vi "__keysight_volatile_test.vi"() -> ()   [LabVIEW 2013]
uses:
  <vilib>/Analysis/NI_AALBase.lvlib
panel:
  out "Numeric":i32
  in  "Frequency Parameters":T1={"Coupling"=TRUE, "Frequency 2 (MHz)"=2.0, "Frequency 1 (MHz)"=2.0} {"Frequency 1 (MHz)" min=0.0 max=14.5; "Frequency 2 (MHz)" min=0.0 max=14.5}
  in  "Array to Binary Block Format 2":dbl[](array[numeric])
  out "concatenated string":string
  out "Waveform Graph":dbl[](graph)
  in  "Pulse Width":i32=1
  in  "N-per-period":i32=20001
  in  "GPIB address of Pulse generator":string="10"
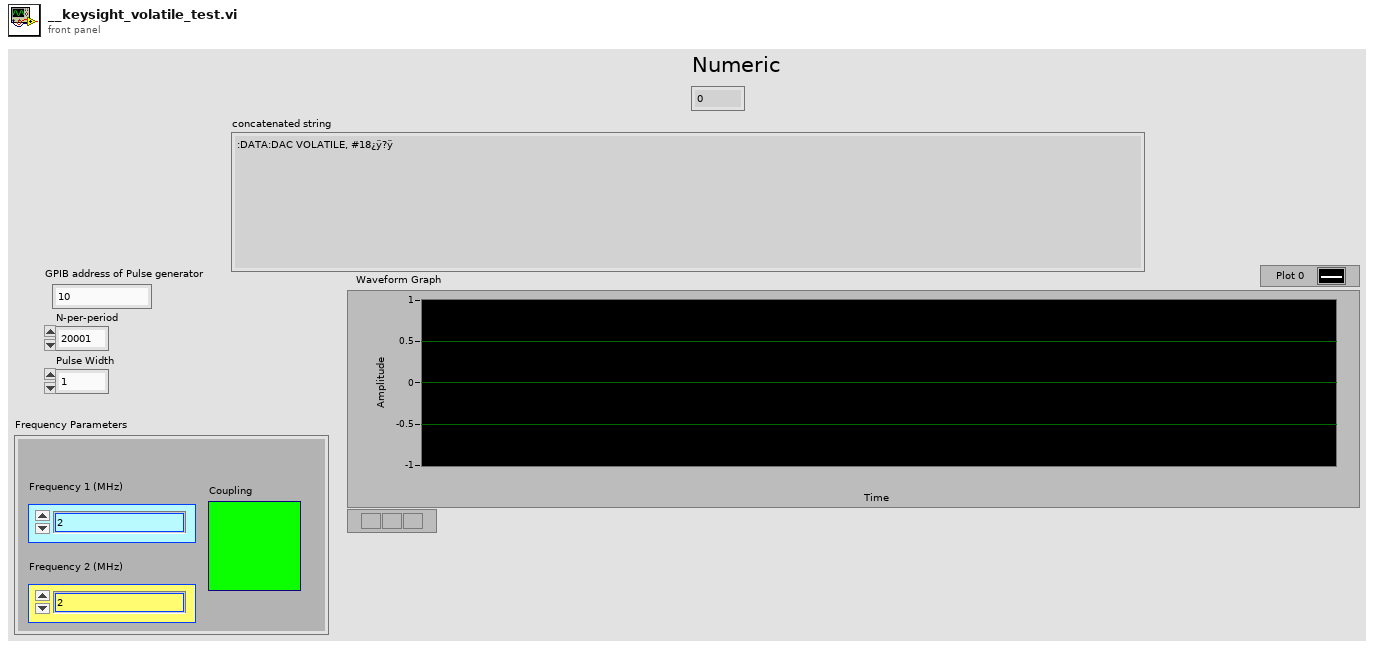
[diagram p1: front panel]
types:
  T1 = cluster{"Coupling":bool, "Frequency 2 (MHz)":dbl, "Frequency 1 (MHz)":dbl}
  T2 = cluster{"Ouput 1":bool, "Ouput 2":bool, "Ouput 1 Neg":bool, "Ouput 2 Neg":bool}
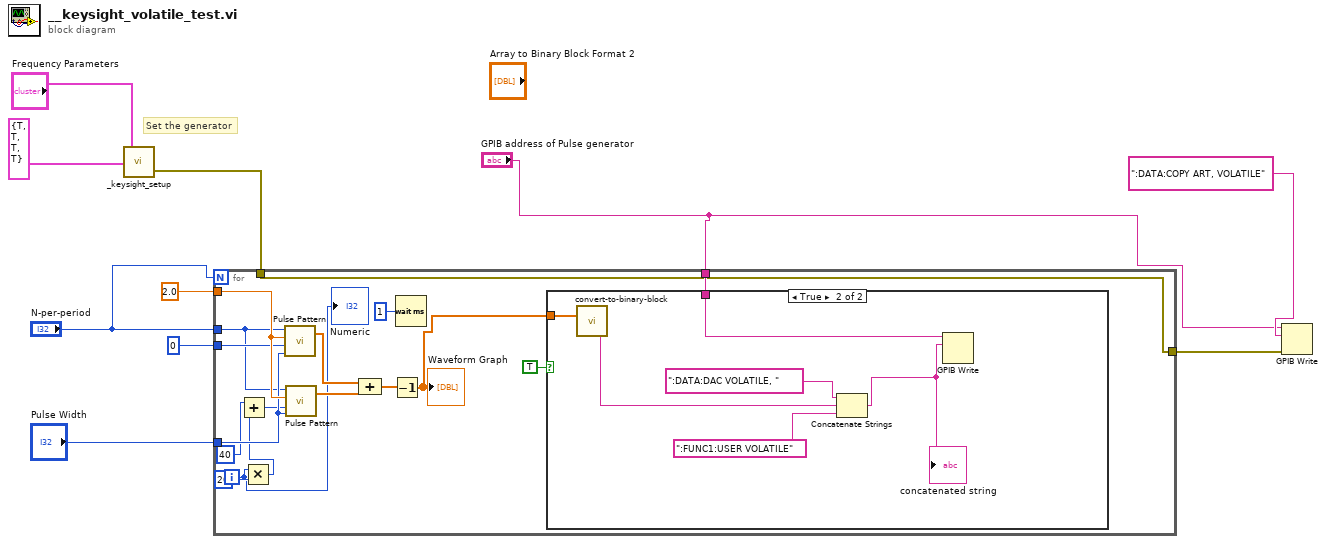
[diagram p0: block diagram]
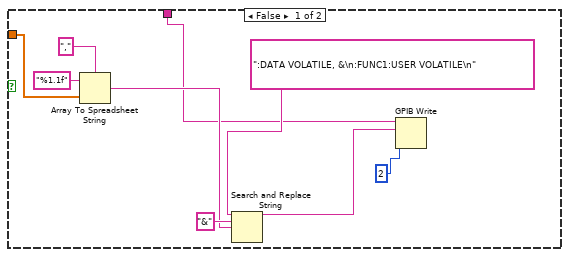
[diagram p2: hidden frame]
diagram:
  # "Set the generator"
  n1 = call "_keysight_setup.vi"("Outputs"=T2 {"Ouput 1"=TRUE, "Ouput 2"=TRUE, "Ouput 1 Neg"=TRUE, "Ouput 2 Neg"=TRUE}, "Frequency Parameters"="Frequency Parameters") -> ("error out"=w7:errorcluster)  [unwired: 1 in, 1 out]
  n2 = for {
    N: "N-per-period" -> [_]
    tunnel: 2.0 -> [w25]
    tunnel: 0 ("delay 2") -> [w24]
    tunnel: "Pulse Width" -> [w23]
    tunnel: "N-per-period" -> [w21]
    tunnel: "GPIB address of Pulse generator" -> [w17]
    tunnel: w7 -> [w16]
    tunnel: [w16] -> w4
    i -> [w11]
    n3 = Multiply(x=w11, y=20) -> (x*y=w12:i32)
    n4 = Add(x=40 ("delay 2"), y=w12) -> (x+y=w18:i32)
    n5 = call <vilib>:"Pulse Pattern.vi"("width"=w23, "delay"=w24, "amplitude"=w25, "samples"=w21) -> ("Pulse Pattern"=w27:dbl[])  [unwired: 1 out]
    n6 = call <vilib>:"Pulse Pattern.vi"("width"=w23, "delay"=w18, "amplitude"=w25, "samples"=w21) -> ("Pulse Pattern"=w26:dbl[])  [unwired: 1 out]
    n7 = Compound Arithmetic op=ADD(w27, w26) -> (w22:dbl[])
    n8 = Decrement(x=w22) -> (x-1=w15:dbl[])
    "Waveform Graph" <- w15
    n9 = Wait (ms)(milliseconds to wait=u32 1) -> ()  [unwired: 1 out]
    n10 = case shown="True" TRUE {
      tunnel: w17 -> [w28 w39]
      tunnel: w15 -> [w34 w37]
      frame False {
        n11 = Array To Spreadsheet String(delimiter (Tab)=",", array=w34, 3:"%1.1f" ("format string")) -> (spreadsheet string=w29:string)
        n12 = Search and Replace String(input string=":DATA VOLATILE, &\n:FUNC1:USER VOLATILE\n", search string="&", replace string=w29) -> (result string=w32:string)  [unwired: 5 in, 3 out]
        n13 = GPIB Write(0:w28, 1:w32, 2:2) -> ()  [unwired: 2 in, 2 out]
      }
      frame True {
        n14 = call "convert-to-binary-block.vi"("Array to Binary Block Format"=w37) -> ("Binary Block"=w41:string)
        n15 = Concatenate Strings(":DATA:DAC VOLATILE, ", w41, ":FUNC1:USER VOLATILE" ("string")) -> (w42:string)
        "concatenated string" <- w42
        n16 = GPIB Write(0:w39, 1:w42) -> ()  [unwired: 3 in, 2 out]
      }
    }
    "Numeric" <- w11
  }
  n17 = GPIB Write(0:"GPIB address of Pulse generator", 1:":DATA:COPY ART, VOLATILE", 3:w4) -> ()  [unwired: 2 in, 2 out]
